vi "Magazine_Test.vi"(11 "Joystick_In":T1) -> ()   [LabVIEW 2019]
uses:
  Utility_VIs/Joystick_Controls.ctl
  Subsystems/Magazine/Magazine_Cluster.ctl
  Globals/Magazine_Globals.vi
panel:
  in  "Magazine_Speed":dbl
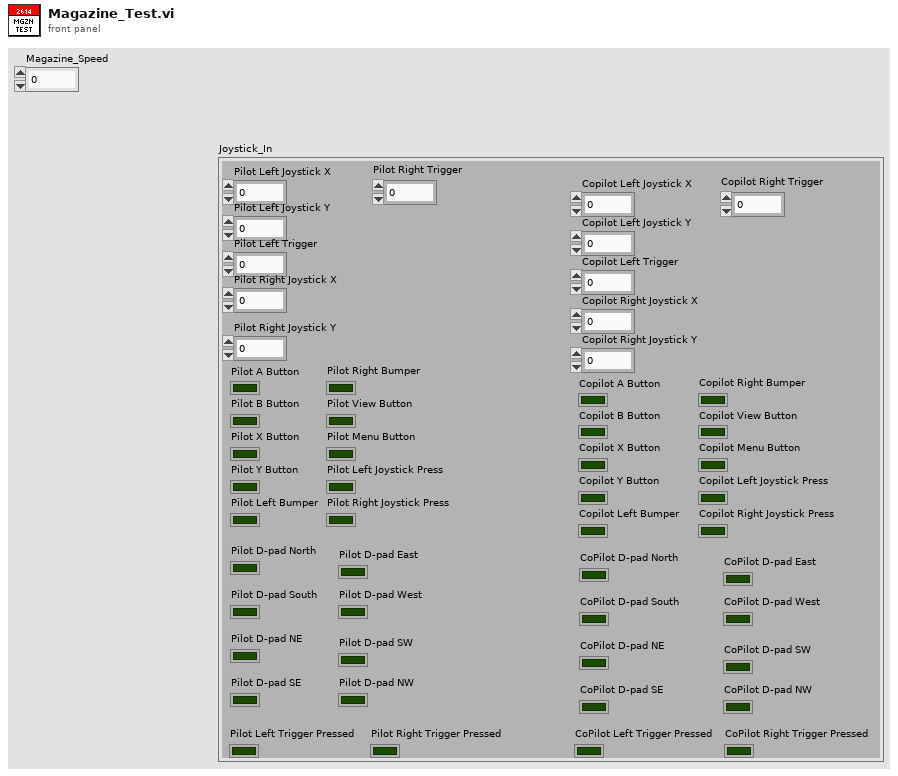
[diagram p1: front panel]
types:
  T1 = typedef "Joystick_Controls.ctl" = cluster{"Pilot Left Joystick X":dbl, "Pilot Left Joystick Y":dbl, "Pilot A Button":bool, "Pilot B Button":bool, "Pilot X Button":bool, "Pilot Y Button":bool, "Pilot Left Bumper":bool, "Pilot Right Bumper":bool, "Pilot View Button":bool, "Pilot Menu Button":bool, "Pilot Left Joystick Press":bool, "Pilot Right Joystick Press":bool, "Pilot Left Trigger":dbl, "Pilot Right Joystick X":dbl, "Pilot Right Joystick Y":dbl, "Pilot Right Trigger":dbl, "Copilot Left Joystick X":dbl, "Copilot Left Joystick Y":dbl, "Copilot A Button":bool, "Copilot B Button":bool, "Copilot X Button":bool, "Copilot Y Button":bool, "Copilot Left Bumper":bool, "Copilot Right Bumper":bool, "Copilot View Button":bool, "Copilot Menu Button":bool, "Copilot Left Joystick Press":bool, "Copilot Right Joystick Press":bool, "Copilot Left Trigger":dbl, "Copilot Right Joystick X":dbl, "Copilot Right Joystick Y":dbl, "Copilot Right Trigger":dbl, "Pilot D-pad North":bool, "Pilot D-pad South":bool, "Pilot D-pad East":bool, "Pilot D-pad West":bool, "Pilot D-pad NE ":bool, "Pilot D-pad SE":bool, "Pilot D-pad SW":bool, "Pilot D-pad NW":bool, "CoPilot D-pad North":bool, "CoPilot D-pad South":bool, "CoPilot D-pad East":bool, "CoPilot D-pad West":bool, "CoPilot D-pad NE":bool, "CoPilot D-pad SE":bool, "CoPilot D-pad SW":bool, "CoPilot D-pad NW":bool, "Pilot Left Trigger Pressed":bool, "Pilot Right Trigger Pressed":bool, "CoPilot Left Trigger Pressed":bool, "CoPilot Right Trigger Pressed":bool}
  T2 = typedef "Magazine_Cluster.ctl" = cluster{"Control_States":enum16{"No-Op", "Loading", "Fire", "Unjam", "Manual"}, "Fire":bool, "Magazine_Throttle":dbl}
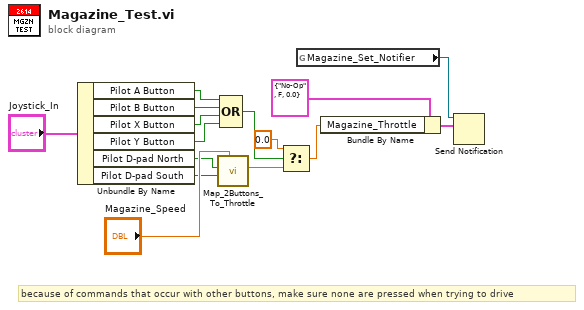
[diagram p0: block diagram]
diagram:
  # "because of commands that occur with other buttons, make sure none are pressed when trying to drive"
  n1 = Unbundle By Name("Joystick_In") -> ("Pilot A Button"=w8:bool, "Pilot B Button"=w7:bool, "Pilot X Button"=w6:bool, "Pilot Y Button"=w5:bool, "Pilot D-pad North"=w10:bool, "Pilot D-pad South"=w9:bool)
  n2 = call "Map_2Buttons_To_Throttle.vi"("Power"="Magazine_Speed", "Down"=w9, "Up"=w10) -> ("Throttle"=w1:dbl)  [unwired: 8 in]
  n3 = Compound Arithmetic op=OR(w8, w7, w6, w5) -> (w3:bool)
  n4 = Select(t=0.0, s=w3, f=w1) -> (s? t:f=w4:dbl)
  n5 = global read "Magazine_Globals.vi" "Magazine_Set_Notifier"() -> (w14:refnum<notifier>)
  n6 = Bundle By Name(cluster=T2 {"Control_States"=enum."No-Op", "Fire"=FALSE, "Magazine_Throttle"=0.0} ("Magazine_Cluster"), "Magazine_Throttle"=w4) -> (w12:T2)
  n7 = Send Notification(notification=w12, notifier=w14) -> ()  [unwired: 1 in, 2 out]
